vi "WLAN_SuperposedFrameBuild - Optimized.vi"(7 "Alpha":dbl min=0.0 max=1.0 step=0.05 format="%#_13g", 8 "error in (no error)":errorcluster, 9 "data in 2":i8[](array[numeric]) caption="input bit stream", 10 "Modulation parameter":T1, 11 "data in":i8[](array[numeric]) caption="input bit stream") -> (0 "error out":errorcluster, 3 "output array":cdb[](array[numeric]))   [LabVIEW 2022 SP3]
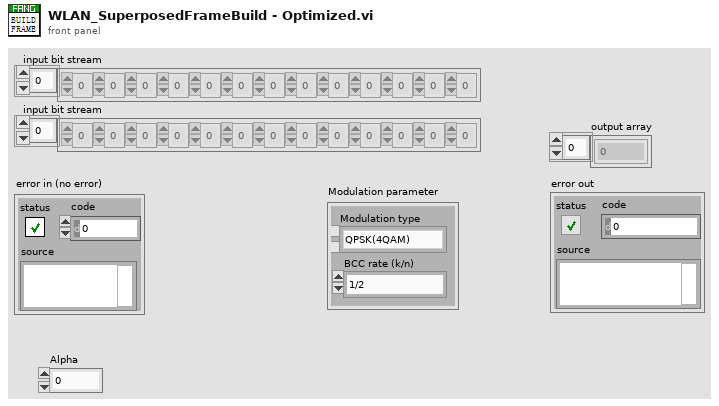
[diagram p1: front panel]
types:
  T1 = cluster{"Modulation type":enum16{"QPSK(4QAM)", "64QAM", "16QAM", "BPSK"}, "BCC rate (k/n)":enum16{"1/2", "2/3", "3/4"}}
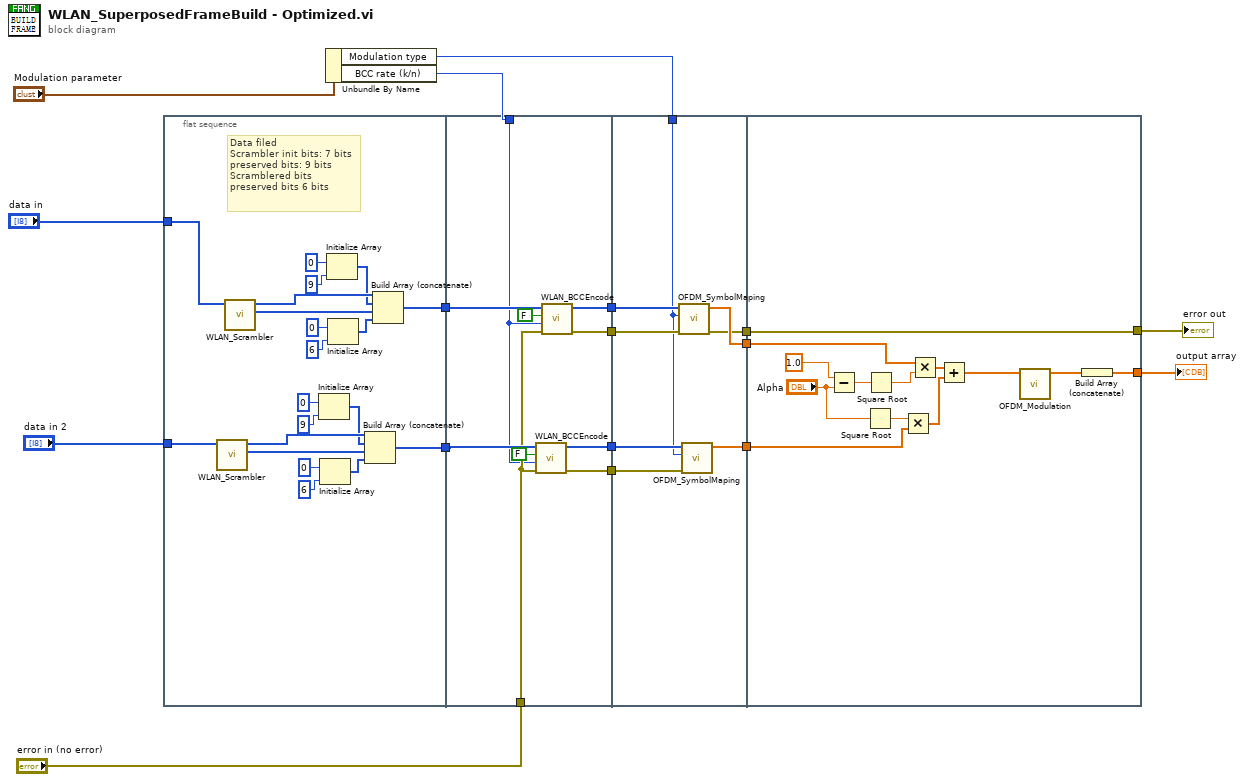
[diagram p0: block diagram]
diagram:
  n1 = flat-sequence {
    tunnel: "data in" -> [w18]
    tunnel: [w30] -> w16
    tunnel: "data in 2" -> [w21]
    tunnel: [w20] -> w5
    tunnel: w16 -> [w44]
    tunnel: "error in (no error)" -> [w40]
    tunnel: [w46] -> w14
    tunnel: [w45] -> w13
    tunnel: w10 -> [w39]
    tunnel: w5 -> [w42]
    tunnel: [w41] -> w4
    tunnel: [w38] -> w3
    tunnel: w14 -> [w55]
    tunnel: w13 -> [w54]
    tunnel: w11 -> [w50]
    tunnel: [w53] -> w9
    tunnel: [w52] -> w8
    tunnel: w4 -> [w51]
    tunnel: w3 -> [w49]
    tunnel: [w48] -> w2
    tunnel: w9 -> [w60]
    tunnel: w8 -> [w57]
    tunnel: [w68] -> w7
    tunnel: w2 -> [w59]
    tunnel: [w57] -> w1
    frame #0 {
      # "Data filed\nScrambler init bits: 7 bits\npreserved bits: 9 bits\nScramblered bits\npreserved bits 6 bits"
      n2 = call "WLAN_Scrambler.vi"("input bit stream"=w21) -> ("scrambled bits"=w25:i8[], "scrambler initial bit"=w29:i8[])  [unwired: 9 in]
      n3 = call "WLAN_Scrambler.vi"("input bit stream"=w18) -> ("scrambled bits"=w19:i8[], "scrambler initial bit"=w37:i8[])  [unwired: 9 in]
      n4 = Initialize Array(i8 0 ("element"), 9 ("dimension size")) -> (w28:i8[])
      n5 = Initialize Array(i8 0 ("element"), 6 ("dimension size")) -> (w22:i8[])
      n6 = Initialize Array(i8 0 ("element"), 9 ("dimension size")) -> (w36:i8[])
      n7 = Initialize Array(i8 0 ("element"), 6 ("dimension size")) -> (w31:i8[])
      n8 = Build Array (concatenate)(w29, w28, w25, w22) -> (w20:i8[])
      n9 = Build Array (concatenate)(w37, w36, w19, w31) -> (w30:i8[])
    }
    frame #1 {
      n10 = call "WLAN_BCCEncode.vi"("error in (no error)"=w40, "BCC rate (k/n)"=w39, "need add zeros?"=FALSE, "input bit stream"=w42) -> ("error out"=w38:errorcluster, "output bit stream 3"=w41:i8[])  [unwired: 6 in]
      n11 = call "WLAN_BCCEncode.vi"("error in (no error)"=w40, "BCC rate (k/n)"=w39, "need add zeros?"=FALSE, "input bit stream"=w44) -> ("error out"=w46:errorcluster, "output bit stream 3"=w45:i8[])  [unwired: 6 in]
    }
    frame #2 {
      n12 = call "OFDM_SymbolMaping.vi"("error in (no error)"=w55, "Modulation type"=w50, "input bit stream"=w54) -> ("error out"=w52:errorcluster, "symbols"=w53:cdb[])  [unwired: 7 in]
      n13 = call "OFDM_SymbolMaping.vi"("error in (no error)"=w49, "Modulation type"=w50, "input bit stream"=w51) -> ("symbols"=w48:cdb[])  [unwired: 7 in, 1 out]
    }
    frame #3 {
      n14 = Subtract(x=1.0, y="Alpha") -> (x-y=w62:dbl)
      n15 = Square Root(x="Alpha") -> (sqrt(x)=w66:dbl)
      n16 = Square Root(x=w62) -> (sqrt(x)=w64:dbl)
      n17 = Multiply(x=w66, y=w59) -> (x*y=w67:cdb[])
      n18 = Multiply(x=w60, y=w64) -> (x*y=w65:cdb[])
      n19 = Add(x=w65, y=w67) -> (x+y=w58:cdb[])
      n20 = call "OFDM_Modulation.vi"("Input sequence"=w58) -> ("Output sequence"=w56:cdb[])  [unwired: 10 in]
      n21 = Build Array (concatenate)(w56) -> (w68:cdb[])
    }
  }
  n22 = Unbundle By Name("Modulation parameter") -> ("Modulation type"=w11:enum16{"QPSK(4QAM)", "64QAM", "16QAM", "BPSK"}, "BCC rate (k/n)"=w10:enum16{"1/2", "2/3", "3/4"})
  "output array" <- w7
  "error out" <- w1
